vi "runTestScenario.vi"(8 "error in (no error)":errorcluster, 11 "Multi Analog Input Voltage Test in":refnum<class "Multi Analog Input Voltage Test.lvclass">) -> (0 "error out":errorcluster, 1 "Result":T1, 2 "TestExecution":T2, 3 "Multi Analog Input Voltage Test out":refnum<class "Multi Analog Input Voltage Test.lvclass">)   [LabVIEW 2015, in "Multi Analog Input Voltage Test.lvclass"]
uses:
  Multi Analog Input Voltage Test.lvclass
  Typedefs/TestExecution.ctl
  Typedefs/PassFailTest.ctl
  Multi Analog Input Voltage Test.lvclass/Multi Analog Input Voltage Test.ctl
  Typedefs/WriteDataFileInput.ctl
  Typedefs/TestScenarioTypes.ctl
  <userlib>/Common/ILC/ILC/ILC.lvclass/ILC.ctl
  Typedefs/WriteLogMessageInput.ctl
  <vilib>/express/express arith-compare/Formula/XNode/ExpressFormulaBlockNode.xnode
  Model/TestLog/ITestLog/ITestLog.lvclass
  Typedefs/ILCBTTypedefs.lvlib
  <userlib>/Common/ILC/ILC/ILC.lvclass
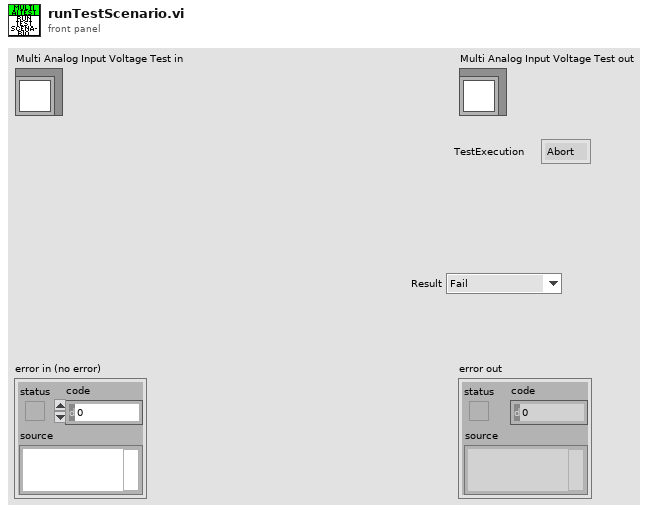
[diagram p1: front panel]
types:
  T1 = typedef "ILCBTTypedefs.lvlib/PassFailTest.ctl" = enum16{"Fail", "Pass", "NA"}
  T2 = typedef "ILCBTTypedefs.lvlib/TestExecution.ctl" = enum16{"Abort", "Continue"}
  T3 = typedef "ILCBTTypedefs.lvlib/TestScenarioTypes.ctl" = enum16{"+3.3VA Supply Test", "+3.3VD Supply Test", "+5VA Supply Test", "+5VD Supply Test", "Unique ID Test", "TEDS Status Test", "LIMSW1_TTL Low Test", "LIMSW1_TTL High Test", "LIMSW2_TTL Low Test", "LIMSW2_TTL High Test", "Tachometer Low Test", "Tachometer High Test", "SSR_TTL Low Test", "SSR_TTL High Test", "SM_GPI Low Test", "SM_GPI High Test", "CW Motion Without Limit Test", "CW Motion With Limit Test", "CW Motion With Both Limits Test", "CW Motion on CCW Limit Test", "CCW Motion Without Limit Test", "CCW Motion With Limit Test", "CCW Motion With Both Limits Test", "CCW Motion on CW Limit Test", "RS232-TXD Low Test", "RS232-TXD High Test", "RS232-RTS Low Test", "RS232-RTS High Test", "RS232-RXD Low Test", "RS232-RXD High Test", "RS232-CTS Low Test", "RS232-CTS High Test", "Out_SS Low Test", "Out_SS High Test", "Out_SDI Low Test", "Out_SDI High Test", "Out_SCLK Low Test", "Out_SCLK High Test", "Reset Low Test", "Reset High Test", "1 Channel ADC Test", "3 Channel ADC Test", "5 Channel ADC Test", "Vref Test", "ROT Test", "DAC1 Test", "DAC2 Test", "DAC3 Test", "DAC4 Test", "BIAS Test", "EXC1 Test", "EXC2 Test", "EXC3 Test", "EXC4 Test"}
  T4 = typedef "ILCBTTypedefs.lvlib/WriteDataFileInput.ctl" = cluster{"Test Scenario":T3, "File Name":string, "Output":string[]}
  T5 = typedef "ILCBTTypedefs.lvlib/WriteLogMessageInput.ctl" = cluster{"Test Scenario":T3, "Description":string, "Actual Value":string, "Data File":string, "Result":T1}
  T6 = typedef "ILCCommon.lvlib/ILCTypedefs.lvlib/InputData.ctl" = cluster{"Input Channels":T7, "Limit Switches":T8, "Tachometer":u16, "SSI Encoder":i32, "ADCs":T9}
  T7 = typedef "ILCCommon.lvlib/ILCConfiguration.lvlib/InputChannels.ctl" = enum16{"Channel 0", "3 Channels", "5 Channels"}
  T8 = typedef "ILCCommon.lvlib/ILCTypedefs.lvlib/LimitSwitches.ctl" = cluster{"1":bool, "2":bool}
  T9 = typedef "ILCCommon.lvlib/ILCTypedefs.lvlib/ADCs.ctl" = cluster{"Ch0":i32, "Ch1":i32, "Ch2":i32, "Ch3":i32, "Ch4":i32}
  T10 = typedef "ILCCommon.lvlib/ILCTypedefs.lvlib/ADCsInEngineeringUnits.ctl" = cluster{"Ch1":dbl, "Ch2":dbl, "Ch3":dbl, "Ch4":dbl}
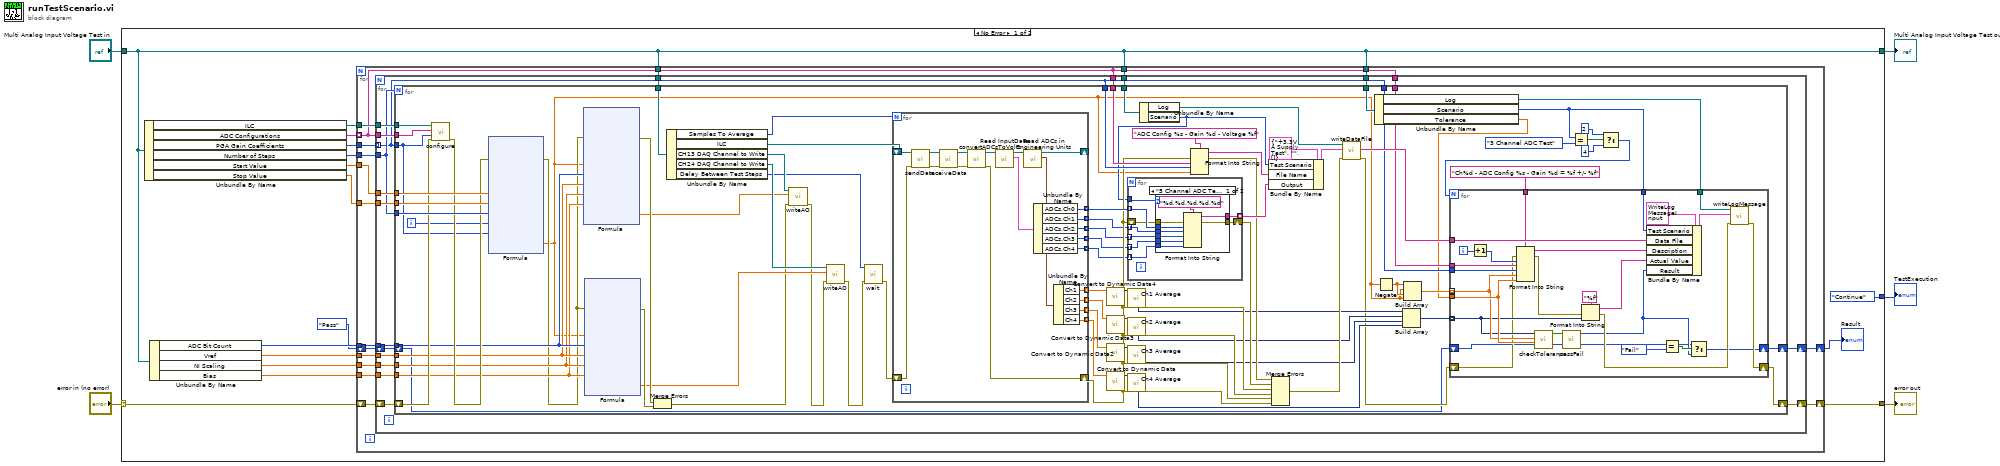
[diagram p0: block diagram]
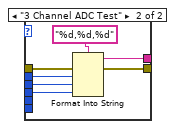
[diagram p2: hidden frame]
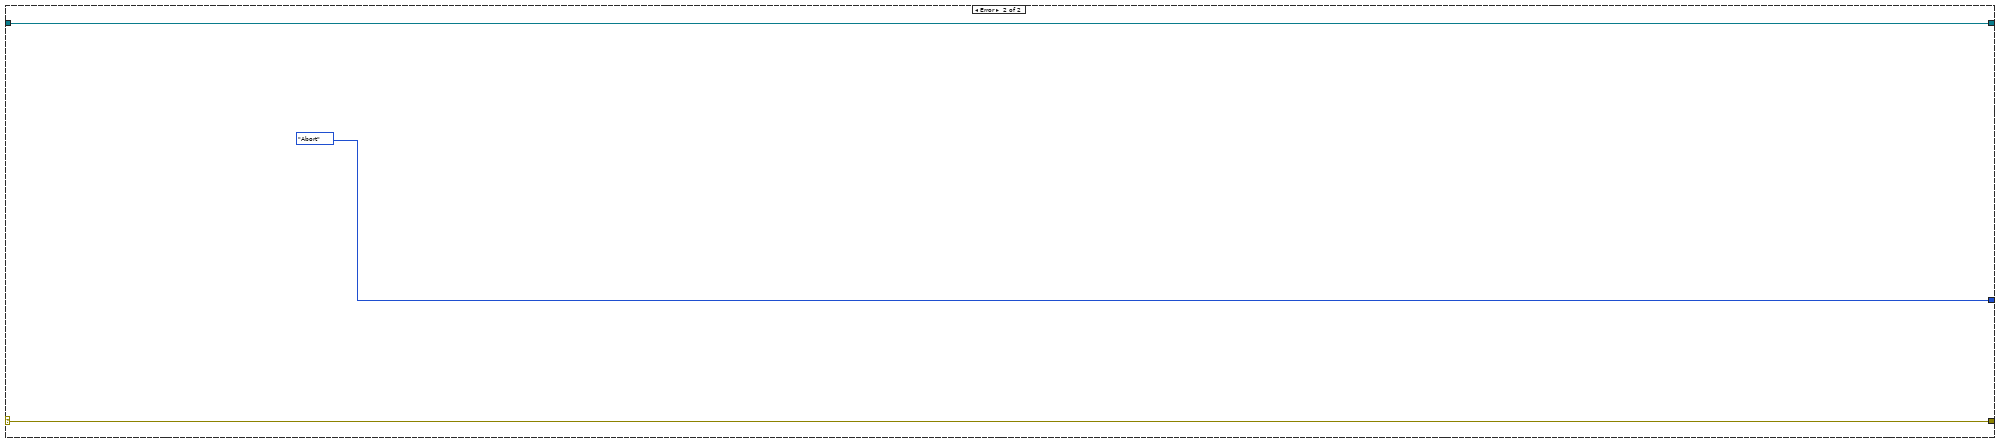
[diagram p3: hidden frame]
diagram:
  n1 = case shown="No Error" "error in (no error)" {
    selector: "error in (no error)" -> [w14 w263]
    tunnel: [w9 w263] -> w4
    tunnel: [w8 w264] -> w3
    tunnel: "Multi Analog Input Voltage Test in" -> [w8 w264]
    tunnel: [TestExecution."Continue" ("TestExecution") TestExecution."Abort" ("TestExecution")] -> w1
    frame No Error {
      n2 = Unbundle By Name(w8) -> ("ILC"=w17:refnum<class "ILC.lvclass">, "ADC Configurations"=w20:string[], "PGA Gain Coefficients"=w19:u16[], "Number of Steps"=w18:u16, "Start Value"=w16:dbl, "Stop Value"=w15:dbl)
      n3 = Unbundle By Name(w8) -> ("ADC Bit Count"=w13:u16, "Vref"=w12:dbl, "NI Scaling"=w11:dbl, "Bias"=w10:dbl)
      n4 = for {
        tunnel: w20 -> [w24] mode=indexing
        tunnel: w19 -> [w38]
        tunnel: w18 -> [w37]
        tunnel: w17 -> [w36]
        tunnel: w16 -> [w35]
        tunnel: w15 -> [w34]
        shift-right: [w32] -> w9
        shift-left: w14 -> [w33]
        tunnel: w13 -> [w31]
        tunnel: w12 -> [w30]
        tunnel: w11 -> [w29]
        tunnel: w10 -> [w28]
        tunnel: w8 -> [w27]
        tunnel: w8 -> [w26]
        tunnel: w8 -> [w25]
        shift-right: [w23] -> w6
        shift-left: PassFailTest."Pass" ("Result") -> [w22]
        n5 = for {
          tunnel: w38 -> [w41] mode=indexing
          tunnel: w37 -> [w53]
          tunnel: w24 -> [w57]
          tunnel: w36 -> [w56]
          tunnel: w35 -> [w55]
          tunnel: w34 -> [w54]
          shift-right: [w51] -> w32
          shift-left: w33 -> [w52]
          tunnel: w31 -> [w50]
          tunnel: w30 -> [w49]
          tunnel: w29 -> [w48]
          tunnel: w28 -> [w47]
          tunnel: w27 -> [w46]
          tunnel: w26 -> [w45]
          tunnel: w24 -> [w44]
          tunnel: w25 -> [w43]
          tunnel: w24 -> [w42]
          shift-right: [w40] -> w23
          shift-left: w22 -> [w39]
          n6 = for {
            N: w53 -> [_]
            tunnel: w57 -> [w140]
            tunnel: w41 -> [w64]
            tunnel: w56 -> [w141]
            tunnel: w55 -> [w139]
            tunnel: w54 -> [w138]
            tunnel: w53 -> [w137]
            shift-right: [w78] -> w51
            shift-left: w52 -> [w136]
            tunnel: w50 -> [w134]
            tunnel: w49 -> [w133]
            tunnel: w48 -> [w132]
            tunnel: w47 -> [w131]
            tunnel: w46 -> [w127]
            tunnel: w45 -> [w118]
            tunnel: w41 -> [w109]
            tunnel: w44 -> [w110]
            tunnel: w43 -> [w105]
            tunnel: w42 -> [w84]
            tunnel: w41 -> [w83]
            shift-right: [w63] -> w40
            shift-left: w39 -> [w62]
            i -> [w66]
            n7 = call <userlib>:"configure.vi"("error in (no error)"=w136, "PGA Gain"=w64, "ADC Configuration"=w140, "ILC in"=w141) -> ("error out"=w135:errorcluster)  [unwired: 6 in, 1 out]
            n8 = xnode "Formula"("START"=w139, "STOP"=w138, "NUM"=w137, "X"=w66, "GAIN"=w64, "error in (no error)"=w135) -> ("Result"=w65:dbl, "error out"=w130:errorcluster)
            n9 = xnode "Formula"("X"=w65, "ADCBITS"=w134, "VREF"=w133, "SCALING"=w132, "BIAS"=w131, "error in (no error)"=w130) -> ("Result"=w124:dbl, "error out"=w129:errorcluster)
            n10 = xnode "Formula"("X"=w65, "ADCBITS"=w134, "VREF"=w133, "SCALING"=w132, "BIAS"=w131, "error in (no error)"=w130) -> ("Result"=w123:dbl, "error out"=w128:errorcluster)
            n11 = Merge Errors(w129, w128) -> (w122:errorcluster)
            n12 = Unbundle By Name(w127) -> ("Samples To Average"=w120:i32, "ILC"=w119:refnum<class "ILC.lvclass">, "CH13 DAQ Channel to Write"=w126:refnum<k21>, "CH24 DAQ Channel to Write"=w125:refnum<k21>, "Delay Between Test Steps"=w69:u16)
            n13 = call "writeAO.vi"("error in (no error)"=w122, "Value"=w124, "DAQ Channel To Write"=w126) -> ("error out"=w121:errorcluster)  [unwired: 8 in]
            n14 = call "writeAO.vi"("error in (no error)"=w121, "Value"=w123, "DAQ Channel To Write"=w125) -> ("error out"=w68:errorcluster)  [unwired: 8 in]
            n15 = call "wait.vi"("error in (no error)"=w68, "Wait Time"=w69) -> ("error out"=w67:errorcluster)  [unwired: 9 in]
            n16 = for {
              N: w120 -> [_]
              tunnel: [w256] -> w96 mode=indexing
              tunnel: [w255] -> w99 mode=indexing
              tunnel: [w254] -> w114 mode=indexing
              tunnel: [w253] -> w101 mode=indexing
              tunnel: [w252] -> w103 mode=indexing
              shift-right: [w251] -> _
              shift-left: w119 -> [w261]
              shift-right: [w246] -> w104
              shift-left: w67 -> [w250]
              tunnel: [w244] -> w61 mode=indexing
              tunnel: [w243] -> w60 mode=indexing
              tunnel: [w242] -> w59 mode=indexing
              tunnel: [w241] -> w58 mode=indexing
              n17 = call <userlib>:"sendData.vi"("error in (no error)"=w250, "ILC in"=w261) -> ("error out"=w249:errorcluster, "ILC out"=w260:refnum<class "ILC.lvclass">)  [unwired: 8 in]
              n18 = call <userlib>:"receiveData.vi"("error in (no error)"=w249, "ILC in"=w260) -> ("error out"=w247:errorcluster, "ILC out"=w248:refnum<class "ILC.lvclass">)  [unwired: 8 in]
              n19 = call <userlib>:"convertADCsToVolts.vi"("error in (no error)"=w247, "ILC in"=w248) -> ("error out"=w246:errorcluster, "ILC out"=w245:refnum<class "ILC.lvclass">)  [unwired: 8 in]
              n20 = call <userlib>:"Read InputData.vi"("ILC in"=w245) -> ("InputData"=w259:T6, "ILC out"=w258:refnum<class "ILC.lvclass">)  [unwired: 9 in]
              n21 = call <userlib>:"Read ADCs in Engineering Units.vi"("ILC in"=w258) -> ("ADCs in Engineering Units"=w257:T10, "ILC out"=w251:refnum<class "ILC.lvclass">)  [unwired: 9 in]
              n22 = Unbundle By Name(w259) -> ("ADCs.Ch0"=w254:i32, "ADCs.Ch1"=w244:i32, "ADCs.Ch2"=w243:i32, "ADCs.Ch3"=w242:i32, "ADCs.Ch4"=w241:i32)
              n23 = Unbundle By Name(w257) -> ("Ch1"=w256:dbl, "Ch2"=w255:dbl, "Ch3"=w253:dbl, "Ch4"=w252:dbl)
            }
            n24 = call "Convert to Dynamic Data4"("Array"=w96) -> ("Dynamic Data Type"=w97:dynamicdata)  [unwired: 3 in]
            n25 = call "Convert to Dynamic Data3"("Array"=w99) -> ("Dynamic Data Type"=w98:dynamicdata)  [unwired: 3 in]
            n26 = call "Convert to Dynamic Data2"("Array"=w101) -> ("Dynamic Data Type"=w100:dynamicdata)  [unwired: 3 in]
            n27 = call "Convert to Dynamic Data"("Array"=w103) -> ("Dynamic Data Type"=w102:dynamicdata)  [unwired: 3 in]
            n28 = call "Ch1 Average"("Signals"=w97, "error in (no error)"=w104) -> ("Arithmetic Mean"=w91:dynamicdata, "error out"=w95:errorcluster)  [unwired: 24 in]
            n29 = call "Ch2 Average"("Signals"=w98, "error in (no error)"=w104) -> ("Arithmetic Mean"=w90:dynamicdata, "error out"=w92:errorcluster)  [unwired: 24 in]
            n30 = call "Ch3 Average"("Signals"=w100, "error in (no error)"=w104) -> ("Arithmetic Mean"=w89:dynamicdata, "error out"=w93:errorcluster)  [unwired: 24 in]
            n31 = call "Ch4 Average"("Signals"=w102, "error in (no error)"=w104) -> ("Arithmetic Mean"=w88:dynamicdata, "error out"=w94:errorcluster)  [unwired: 24 in]
            n32 = Unbundle By Name(w118) -> ("Log"=w117:refnum<class "ITestLog.lvclass">, "Scenario"=w70:T3)
            n33 = for {
              tunnel: w114 -> [w220] mode=indexing
              tunnel: w61 -> [w221] mode=indexing
              tunnel: w60 -> [w222] mode=indexing
              tunnel: w59 -> [w223] mode=indexing
              tunnel: w58 -> [w224] mode=indexing
              tunnel: [w219] -> w113 mode=indexing
              shift-right: [w217] -> w107
              shift-left: w104 -> [w218]
              tunnel: w70 -> [w216]
              n34 = case shown="\"5 Channel ADC Test\", Default" w216 {
                tunnel: w224 -> [w232 _]
                tunnel: w223 -> [w231 _]
                tunnel: w222 -> [w230 w239]
                tunnel: w221 -> [w229 w238]
                tunnel: w220 -> [w228 w237]
                tunnel: [w227 w236] -> w219
                tunnel: w218 -> [w226 w235]
                tunnel: [w225 w234] -> w217
                frame "5 Channel ADC Test", Default {
                  n35 = Format Into String(format string="%d,%d,%d,%d,%d", error in=w226, w228, w229, w230, w231, w232) -> (resulting string=w227:string, error out=w225:errorcluster)  [unwired: 1 in]
                }
                frame "3 Channel ADC Test" {
                  n36 = Format Into String(format string="%d,%d,%d", error in=w235, w237, w238, w239) -> (resulting string=w236:string, error out=w234:errorcluster)  [unwired: 1 in]
                }
              }
            }
            n37 = Format Into String(format string="ADC Config %s - Gain %d - Voltage %f", error in=w104, w110, w109, w65) -> (resulting string=w111:string, error out=w108:errorcluster)  [unwired: 1 in]
            n38 = Bundle By Name(cluster=T4 {"Test Scenario"=enum."+3.3VA Supply Test", "File Name"="", "Output"=[]} ("WriteDataFileInput"), "Test Scenario"=w70, "File Name"=w111, "Output"=w113) -> (w115:T4)
            n39 = Merge Errors(w108, w107, w95, w92, w93, w94) -> (w106:errorcluster)
            n40 = call-dynamic "writeDataFile.vi"("error in (no error)"=w106, "WriteDataFileInput"=w115, "ITestLog in"=w117) -> ("error out"=w79:errorcluster, "Relative Path"=w86:string)  [unwired: 6 in, 1 out]
            n41 = Unbundle By Name(w105) -> ("Log"=w87:refnum<class "ITestLog.lvclass">, "Scenario"=w76:T3, "Tolerance"=w81:dbl)
            n42 = Negate(x=w65) -> (-x=w77:dbl)
            n43 = Build Array(w91, w90, w89, w88) -> (w80:dynamicdata[])
            n44 = Build Array(w77, w65, w77, w65) -> (w82:dbl[])
            n45 = Equal?(x=w76, y=TestScenarioTypes."3 Channel ADC Test") -> (x = y?=w74:bool)
            n46 = Select(t=2, s=w74, f=4) -> (s? t:f=w71:i32)
            n47 = for {
              N: w71 -> [_]
              tunnel: w76 -> [w213]
              tunnel: w87 -> [w212]
              tunnel: w86 -> [w211]
              tunnel: "Ch%d - ADC Config %s - Gain %d = %f +/- %f" ("format string") -> [w207]
              tunnel: w84 -> [w204]
              tunnel: w83 -> [w203]
              tunnel: w82 -> [w201] mode=indexing
              tunnel: w81 -> [w202]
              tunnel: w80 -> [w200] mode=indexing
              shift-right: [w195] -> w78
              shift-left: w79 -> [w198]
              shift-right: [w191] -> w63
              shift-left: w62 -> [w190]
              i -> [w206]
              n48 = Increment(x=w206) -> (x+1=w205:i32)
              n49 = Format Into String(format string=w207, error in=w198, w205, w204, w203, w201, w202) -> (resulting string=w199:string, error out=w197:errorcluster)  [unwired: 1 in]
              n50 = call "checkTolerance.vi"("Tolerance"=w202, "Expected Value"=w201, "Average"=w200) -> ("Boolean"=w210:bool)  [unwired: 8 in]
              n51 = call "passFail.vi"("Boolean"=w210) -> ("Result"=w192:T1)  [unwired: 10 in]
              n52 = Format Into String(format string="%f", error in=w197, w200) -> (resulting string=w208:string, error out=w196:errorcluster)  [unwired: 1 in]
              n53 = Bundle By Name(cluster=T5 {"Test Scenario"=enum."+3.3VA Supply Test", "Description"="", "Actual Value"="", "Data File"="", "Result"=enum."Fail"} ("WriteLogMessageInput"), "Test Scenario"=w213, "Data File"=w211, "Description"=w199, "Actual Value"=w208, "Result"=w192) -> (w215:T5)
              n54 = Equal?(x=w190, y=PassFailTest."Fail") -> (x = y?=w193:bool)
              n55 = Select(t=w190, s=w193, f=w192) -> (s? t:f=w191:T1)
              n56 = call-dynamic "writeLogMessage.vi"("error in (no error)"=w196, "WriteLogMessageInput"=w215, "ITestLog in"=w212) -> ("error out"=w195:errorcluster)  [unwired: 7 in, 1 out]
            }
          }
        }
      }
      "Result" <- w6
    }
    frame Error {
    }
  }
  "error out" <- w4
  "Multi Analog Input Voltage Test out" <- w3
  "TestExecution" <- w1
